vi "WriteItems.vi"(4 "Items":T1[](array[typedef]), 5 "section":string, 6 "error in":errorcluster, 9 "Path":path) -> (0 "error out":errorcluster)   [LabVIEW 2014, in "PythonConfiguration.lvclass"]
uses:
  PythonConfiguration.lvclass
  TypeDefs/ItemTD.ctl
  <vilib>/Utility/config.llb/NI_LVConfig.lvlib
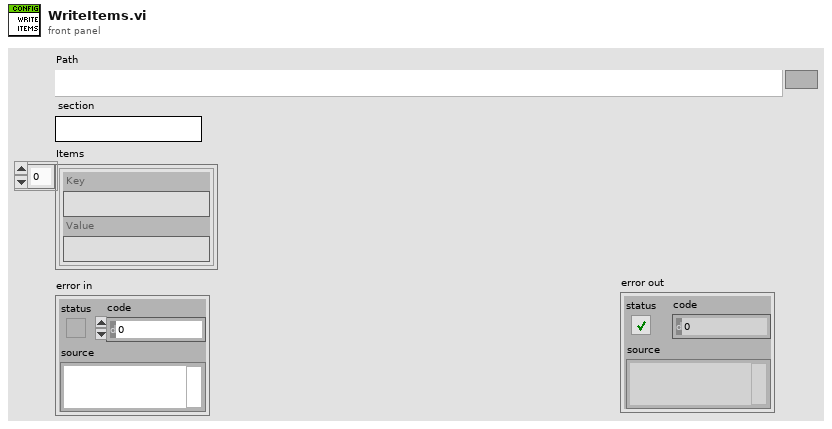
[diagram p1: front panel]
types:
  T1 = typedef "PythonConfiguration.lvclass/ItemTD.ctl" = cluster{"Key":string, "Value":string}
  T2 = typedef "NI_LVConfig.lvlib/Config Data RefNum.ctl" = refnum<k1>
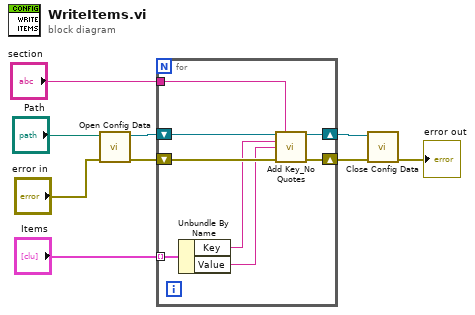
[diagram p0: block diagram]
diagram:
  n1 = call <vilib>:"Open Config Data.vi"("error in (no error)"="error in", "configuration file path"="Path") -> ("error out"=w6:errorcluster, "refnum"=w7:T2)  [unwired: 7 in, 1 out]
  n2 = for {
    shift-right: [w16] -> w3
    shift-left: w7 -> [w13]
    shift-right: [w15] -> w2
    shift-left: w6 -> [w14]
    tunnel: "Items" -> [w17] mode=indexing
    tunnel: "section" -> [w12]
    n3 = Unbundle By Name(w17) -> ("Key"=w11:string, "Value"=w10:string)
    n4 = call "Add Key_No Quotes.vi"("refnum"=w13, "section"=w12, "key"=w11, "value"=w10, "error in (no error)"=w14) -> ("refnum out"=w16:T2, "error out"=w15:errorcluster)  [unwired: 8 in, 1 out]
  }
  n5 = call <vilib>:"Close Config Data.vi"("error in (no error)"=w2, "refnum"=w3) -> ("error out"=→"error out":errorcluster)  [unwired: 8 in, 1 out]
